vi "StringTag.lookup_lua.vi"(5 "LuaVIEW reference":T1) -> (15 "error out":errorcluster)   [LabVIEW 2012]
doc: "Looks up the string tag with the provided name in the collection of live tags and returns a new tag object that allows that tag to be operated upon. This function is typically called in the initialisation section of a script for all required tags so as to ensure that the script fails at an early stage when not all these tags exist.\n\nSince tag names are guaranteed to be valid Lua identifiers, it is possible to assign the returned object to a variable with the same name as the tag. This is <b>not</b> advisable when the tag might change, or it is likely that a copy of the script will be made to serve a different set of tags, since then the script would have to be changed in multiple places (to keep the tag name and various uses of the object variable mutually consistent) instead of just a single place. In such cases it is better to use a short generic variable name, or a name that reflects the role of the tag in the context of the script's actions.\nParameters:\nstr:name, name of the string tag for which to return an object.\nResults:\nobj:strtag, LuaVIEW object referencing the specified string tag.\nErrors:\nNo live tag with the provided name exists.\nSpecified tag is not a string tag.\nData logger not initialized."
uses:
  luaview/typedefs/t_LuaVIEW Reference.ctl
  typedefs/t_DataLog Tag Hash Methods.ctl
  typedefs/t_DataLog Tag Info List Methods.ctl
  luaview/subvis/private/LuaVIEW Pull (string).vi
  luaview/subvis/private/LuaVIEW Push (object).vi
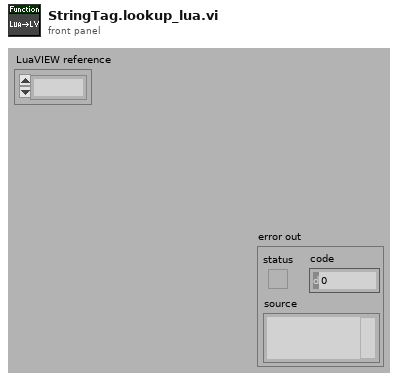
[diagram p1: front panel]
types:
  T1 = typedef "t_LuaVIEW Reference.ctl" = refnum<k1>
  T2 = typedef "t_DataLog Tag Info List Methods.ctl" = enum16{"initialize", "create", "create empty", "rename", "delete", "test tag", "get", "get by name", "get default", "get list", "get path", "get subsets", "set subsets", "set config", "set capacity", "#tags", "go live", "set unlocked", "set mirrored"}
  T3 = typedef "t_DataLog Tag Hash Methods.ctl" = enum16{"initialize", "add tag", "index tag", "lookup", "#tags", "cleanup", "write recovery", "read recovery", "delete recovery"}
  T4 = typedef "t_DataLog Tag Config.ctl" = cluster{"name":string, "unit":string, "temporal":T5, "value":T6, "index":i32, "capacity":i32, "is meta?":bool, "mincapacity":i32, "deadband":dbl, "limit delay":dbl, "format":T7, "precision":u8, "undefine":bool, "update":bool, "update period":u16, "expression":string, "description":string, "logging algorithm":T8, "logging parameters":dbl[]}
  T5 = typedef "t_DataLog Temporal Types.ctl" = enum16{"set&hold", "sample", "event"}
  T6 = typedef "t_DataLog Value Types.ctl" = enum16{"number", "string"}
  T7 = typedef "t_DataLog Numerical Format.ctl" = enum8{"fractional", "exponential", "engineering"}
  T8 = typedef "t_DataLog Logging Algorithms.ctl" = enum16{"nothing", "changes", "everything", "every Nth", "time threshold", "value threshold + prior", "t or v threshold", "t or v threshold + prior"}
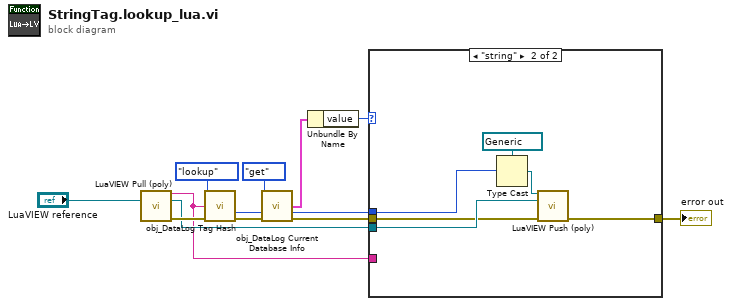
[diagram p0: block diagram]
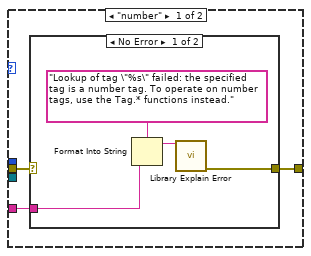
[diagram p2: hidden frame]
diagram:
  n1 = call-poly "LuaVIEW Pull (poly).vi"("LuaVIEW reference in"="LuaVIEW reference") -> ("string"=w2:string, "LuaVIEW reference out"=w3:T1, "error out"=w11:errorcluster)  [unwired: 12 in]
  n2 = call "obj_DataLog Tag Hash.vi"("method"=t_DataLog_Tag_Hash_Methods."lookup", "tag in"=w2, "error in (no error)"=w11) -> ("tag index out"=w8:i32, "error out"=w9:errorcluster)  [unwired: 9 in, 2 out]
  n3 = call "obj_DataLog Current Database Info.vi"("method"=t_DataLog_Tag_Info_List_Methods."get", "tag index/change#"=w8, "error in (no error)"=w9) -> ("tag config out"=w5:T4, "dup tag index"=w7:i32, "error out"=w4:errorcluster)  [unwired: 6 in, 4 out]
  n4 = Unbundle By Name(w5) -> ("value"=w1:T6)
  n5 = case shown="\"string\"" w1 {
    tunnel: [w16 w22] -> w10
    tunnel: w7 -> [_ w25]
    tunnel: w4 -> [w15 w23]
    tunnel: w3 -> [_ w24]
    tunnel: w2 -> [w14 _]
    frame "number" {
      n6 = case shown="No Error" w15 {
        selector: w15 -> [_ w21]
        tunnel: [w17 w21] -> w16
        tunnel: w14 -> [w18 _]
        frame No Error {
          n7 = Format Into String(format string="Lookup of tag \"%s\" failed: the specified tag is a number tag. To operate on number tags, use the Tag.* functions instead." ("string"), w18) -> (resulting string=w20:string)  [unwired: 2 in, 1 out]
          n8 = call "Library Explain Error.vi"("explanation prefix (none)"=w20) -> ("explained error"=w17:errorcluster)  [unwired: 14 in]
        }
        frame Error {
        }
      }
    }
    frame "string" {
      n9 = Type Cast(type=refnum<vi> refnum ("object refnum"), x=w25) -> (*(type *) &x=w26:refnum<vi>)
      n10 = call-poly "LuaVIEW Push (poly).vi"("object refnum"=w26, "LuaVIEW reference in"=w24, "error in (no error)"=w23) -> ("error out"=w22:errorcluster)  [unwired: 11 in, 1 out]
    }
  }
  "error out" <- w10
